vi "Test.vi"() -> ()   [LabVIEW 2016]
uses:
  <vilib>/rvi/DataTransferAndStorage/Container/XNode/niFpgaContainer.xnode
  <vilib>/rvi/Memory/Memory_Emulation/niFpgaMemoryEmulationRefIn.vi
  <userlib>/_NI FLP Library/FPGA/outsideSCTL/FlpLib Multiply Shared Instance 1.vi
  <userlib>/_NI FLP Library/FPGA/outsideSCTL/FlpLib Add Shared Instance 1.vi
panel:
  out "Array":sgl[](array[numeric])
  in  "MatrixSize":i16
  in  "InputMatrixSize":i16
  in  "Matrix":refnum<k21>="DisplacementInputMatrix"
  in  "InputMatrix":refnum<k21>="DisplacementInputMatrix"
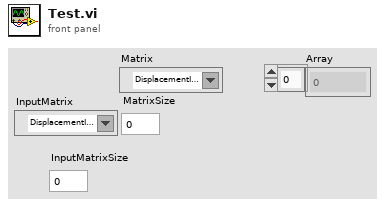
[diagram p1: front panel]
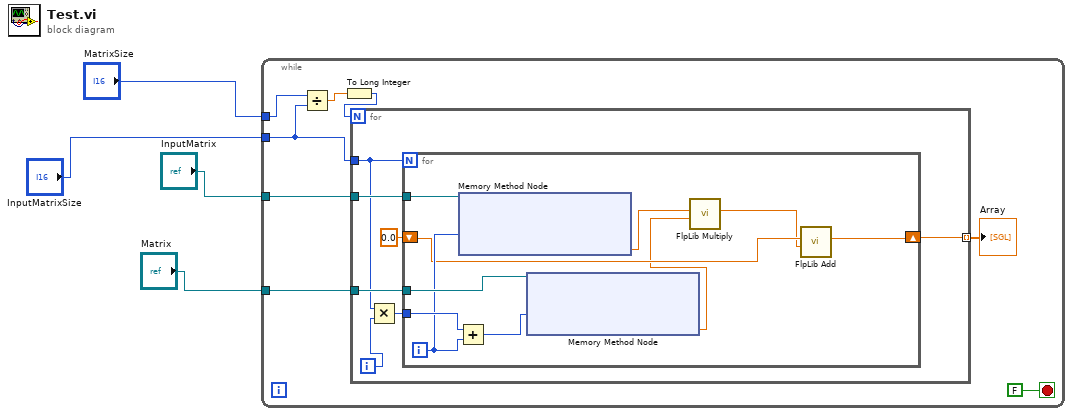
[diagram p0: block diagram]
diagram:
  n1 = while {
    tunnel: "InputMatrix" -> [w12]
    tunnel: "Matrix" -> [w11]
    tunnel: "InputMatrixSize" -> [w9]
    tunnel: "MatrixSize" -> [w10]
    stop <- FALSE stop-if-true
    n2 = Divide(x=w10, y=w9) -> (x/y=w8:dbl)
    n3 = To Long Integer(number=w8) -> (32bit integer=w7:i32)
    n4 = for {
      N: w7 -> [_]
      tunnel: w12 -> [w19]
      tunnel: w11 -> [w18]
      tunnel: w9 -> [w16]
      tunnel: [w13] -> w6 mode=indexing
      i -> [w17]
      n5 = Multiply(x=w16, y=w17) -> (x*y=w15:i32)
      n6 = for {
        N: w16 -> [_]
        tunnel: w19 -> [w29]
        tunnel: w18 -> [w28]
        tunnel: w15 -> [w27]
        shift-right: [w23] -> w13
        shift-left: sgl 0.0 -> [w24]
        i -> [w26]
        n7 = Add(x=w27, y=w26) -> (x+y=w25:i32)
        n8 = xnode ("Memory Method Node")("Address"=w26, "Memory In"=w29) -> ("Data"=w22:sgl)  [unwired: 1 out]
        n9 = xnode ("Memory Method Node")("Address"=w25, "Memory In"=w28) -> ("Data"=w21:sgl)  [unwired: 1 out]
        n10 = call-poly <userlib>:"FlpLib Multiply.vi"("y"=w21, "x"=w22) -> ("x*y"=w20:sgl)  [unwired: 5 in]
        n11 = call-poly <userlib>:"FlpLib Add.vi"("y"=w20, "x"=w24) -> ("x+y"=w23:sgl)  [unwired: 5 in]
      }
    }
    "Array" <- w6
  }
